vi "SecurityUserInterface.vi"() -> ()   [LabVIEW 2023]
uses:
  Control 2.ctl
  <vilib>/Utility/file.llb/Read Delimited Spreadsheet (string).vi
  <vilib>/Utility/file.llb/Write Delimited Spreadsheet (string).vi
  <vilib>/regexp/Match Regular Expression.xnode
panel:
  in  "LogfileUI":enum32{"Page 1"}(tab)
  out "Table Control":string[][](table)
  in  "LoginMenu":enum32{"Page 1", "Page 2"}(tab)
  in  "OK Button":bool
  in  "Username":string
  in  "Password":string
  out "Current Date & Time":string
  in  "ServerUI":enum32{"Page 2"}(tab)
  in  "Logout":bool
  in  "View Log File":bool
  out "Status1":bool
  out "Status2":bool
  out "Status3":bool
  out "Status4":bool
  out "Status5":bool
  out "Status6":bool
  out "Alarm1":bool
  out "Bypass1":bool
  out "Tamper1":bool
  out "Alarm2":bool
  out "Bypass2":bool
  out "Tamper2":bool
  out "Alarm3":bool
  out "Bypass3":bool
  out "Tamper3":bool
  out "Alarm4":bool
  out "Bypass4":bool
  out "Tamper4":bool
  out "Alarm5":bool
  out "Bypass5":bool
  out "Tamper5":bool
  out "Alarm6":bool
  out "Bypass6":bool
  out "Tamper6":bool
  # "Zone Status Log File"
  # "Login Menu"
  # "Zone Status Indicators Panel"
  # "Green = Normal     Red = Alarm       \nOrange = Tamper   Blue = Bypass"
  # "Zone 1"
  # "Zone 2"
  # "Zone 3"
  # "Zone 4"
  # "Zone 5"
  # "Zone 6"
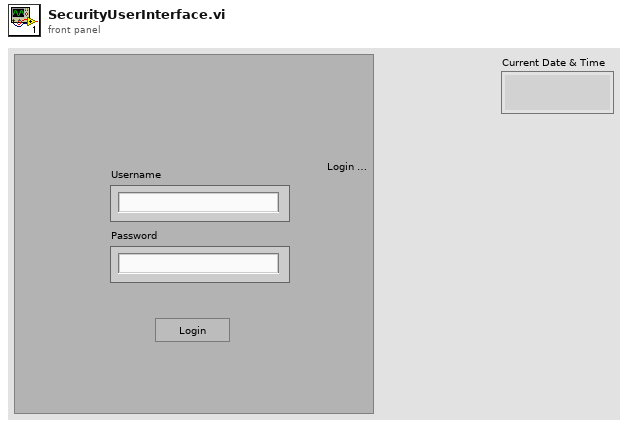
[diagram p1: front panel]
types:
  T1 = typedef "Control 2.ctl" = enum16{"Init", "Wait", "Login", "Logout", "End"}
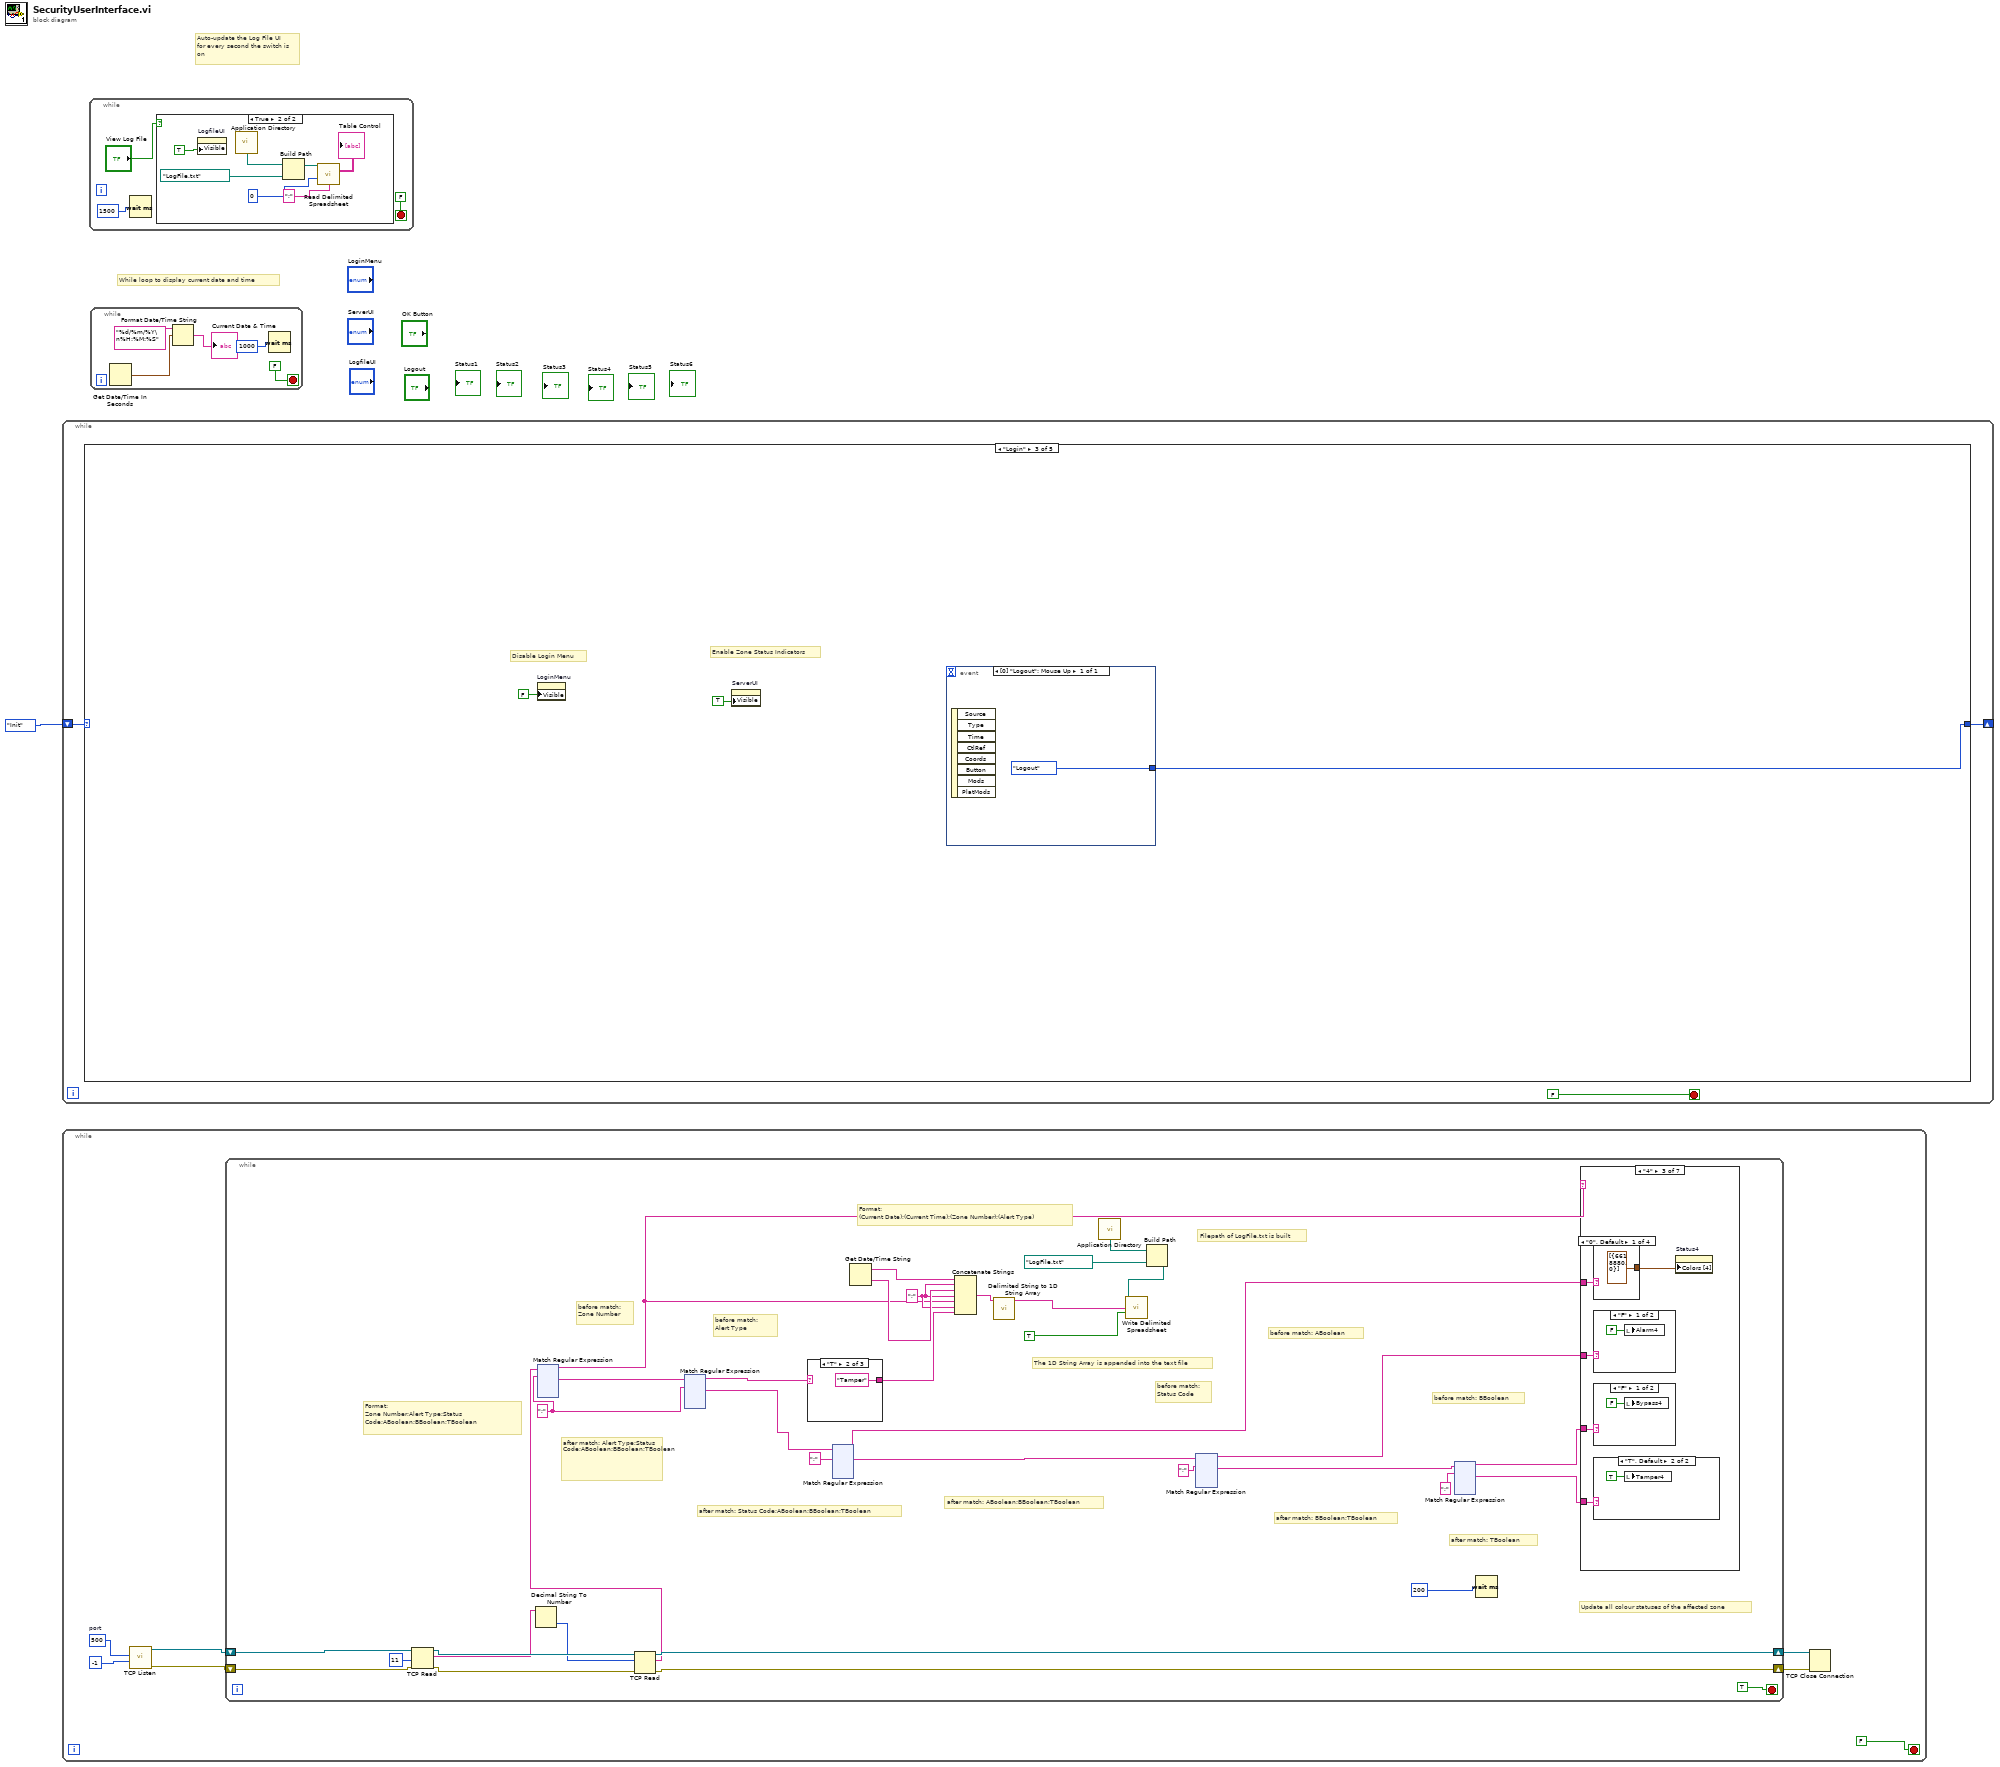
[diagram p0: block diagram]
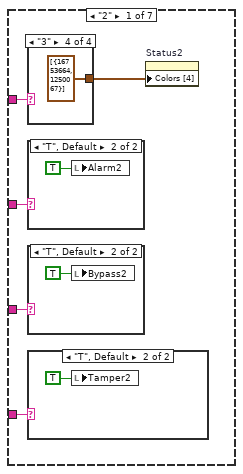
[diagram p2: hidden frame]
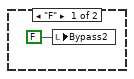
[diagram p3: hidden frame]
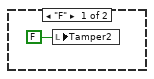
[diagram p4: hidden frame]
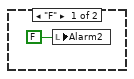
[diagram p5: hidden frame]
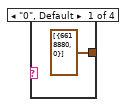
[diagram p6: hidden frame]
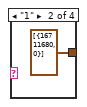
[diagram p7: hidden frame]
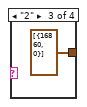
[diagram p8: hidden frame]
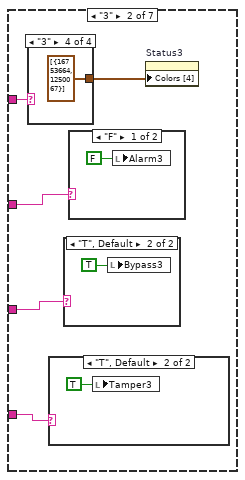
[diagram p9: hidden frame]
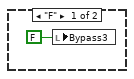
[diagram p10: hidden frame]
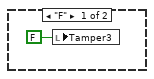
[diagram p11: hidden frame]
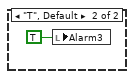
[diagram p12: hidden frame]
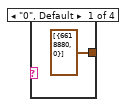
[diagram p13: hidden frame]
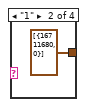
[diagram p14: hidden frame]
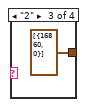
[diagram p15: hidden frame]
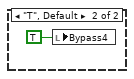
[diagram p16: hidden frame]
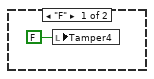
[diagram p17: hidden frame]
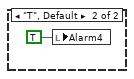
[diagram p18: hidden frame]
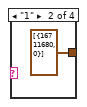
[diagram p19: hidden frame]
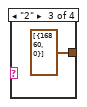
[diagram p20: hidden frame]
diagram:
  # "Auto-update the Log File UI for every second the switch is on"
  # "While loop to display current date and time"
  n1 = while {
    shift-right: [w2] -> _
    shift-left: Control_2."Init" -> [w3]
    stop <- FALSE stop-if-true
    n2 = case shown="\"Login\"" w3 {
      tunnel: [Control_2."Wait" w13 w48 Control_2."Init" Control_2."Init"] -> w2
      frame "Init", Default {
        w8 = cluster{u32, u32}[] [{6618880, 0}] ("Colors [4]")
        w9 = FALSE
        w11 = ""
        # "Enable the Login UI"
        # "Turn off all zone alert LEDs"
        # "Disable Log File Panel"
        # "Initialize all zone statuses to normal state"
        # "Disable Indicator Panel"
        # "Clear Username and Password fields"
        n3 = property on="ServerUI" class="TabCtl (strict)"("Visible"=FALSE) -> ()  [unwired: 2 in, 2 out]
        n4 = property on="LoginMenu" class="TabCtl (strict)"("Visible"=TRUE) -> ()  [unwired: 2 in, 2 out]
        n5 = local write "View Log File"(FALSE ("View Log File")) -> ()
        n6 = local write "Username"(w11) -> ()
        n7 = local write "Password"(w11) -> ()
        n8 = property on="LogfileUI" class="TabCtl (strict)"("Visible"=FALSE) -> ()  [unwired: 2 in, 2 out]
        n9 = property on="Status1" class="Bool (strict)"("Colors [4]"=w8) -> ()  [unwired: 2 in, 2 out]
        n10 = property on="Status2" class="Bool (strict)"("Colors [4]"=w8) -> ()  [unwired: 2 in, 2 out]
        n11 = property on="Status3" class="Bool (strict)"("Colors [4]"=w8) -> ()  [unwired: 2 in, 2 out]
        n12 = property on="Status4" class="Bool (strict)"("Colors [4]"=w8) -> ()  [unwired: 2 in, 2 out]
        n13 = property on="Status5" class="Bool (strict)"("Colors [4]"=w8) -> ()  [unwired: 2 in, 2 out]
        n14 = property on="Status6" class="Bool (strict)"("Colors [4]"=w8) -> ()  [unwired: 2 in, 2 out]
        "Alarm1" <- w9
        "Bypass1" <- w9
        "Tamper1" <- w9
        "Tamper2" <- w9
        "Tamper3" <- w9
        "Tamper4" <- w9
        "Tamper5" <- w9
        "Tamper6" <- w9
        "Alarm4" <- w9
        "Bypass4" <- w9
        "Alarm5" <- w9
        "Bypass5" <- w9
        "Alarm6" <- w9
        "Bypass6" <- w9
        "Alarm3" <- w9
        "Bypass3" <- w9
        "Bypass2" <- w9
        "Alarm2" <- w9
      }
      frame "Wait" {
        n15 = event shown="[0] \"OK Button\": Mouse Up" {
          selector: _ -> [_]
          dyn-events: _ -> [_]
          timeout: _ -> [_]
          tunnel: [w20] -> w13
          event "OK Button": Mouse Up {
            # "Decrement"
            # "Filepath of Users.txt is built"
            # "Array indexing ensures that a username cannot use the password of another user"
            # "Gets an array of usernames"
            # "Gets an array of passwords"
            # "Reads all rows of the Users.txt file into a spreadsheet format with the delimiter ;"
            # "Stops the while loop when it reaches the end of the file, or a matching username has been found"
            n16 = event-data() -> ()  [unwired: 1 in, 8 out]
            n17 = call <vilib>:"Application Directory.vi"() -> ("Application Directory"=w27:path)
            n18 = Build Path(base path=w27, name or relative path="Users.txt") -> (appended path=w26:path)
            n19 = call-poly <vilib>:"Read Delimited Spreadsheet.vi"("file path (dialog if empty)"=w26, "delimiter (\\t)"=";" ("delimiter (\\t)")) -> ("all rows"=w25:string[][])  [unwired: 8 in, 5 out]
            n20 = Index Array "Index Array"(array=w25, index (col)=0) -> (element=w19:string[])  [unwired: 1 in]
            n21 = Array Size(array=w19) -> (size(s)=w18:i32)
            n22 = Index Array "Index Array"(array=w25, index (col)=1) -> (element=w24:string[])  [unwired: 1 in]
            n23 = Decrement(x=w18) -> (x-1=w17:i32)
            n24 = while {
              tunnel: w19 -> [w37] mode=indexing
              tunnel: "Username" -> [w36]
              tunnel: "Password" -> [w35]
              tunnel: w24 -> [w34] mode=indexing
              tunnel: [w33] -> w20
              tunnel: w17 -> [w31]
              i -> [w32]
              stop <- w28 stop-if-true
              n25 = Equal?(x=w36, y=w37) -> (x = y?=w30:bool)
              n26 = Equal?(x=w32, y=w31) -> (x = y?=w29:bool)
              n27 = Or(x=w30, y=w29) -> (x .or. y?=w28:bool)
              n28 = case shown="True" w30 {
                tunnel: w35 -> [_ w42]
                tunnel: w34 -> [_ w43]
                tunnel: [Control_2."Login" w40] -> w33
                frame False {
                  # "When there is no matching username, clear the username field and go back to login"
                  n29 = local write "Username"("") -> ()
                }
                frame True {
                  # "When a matching username is found, check for its corresponding password"
                  n30 = Equal?(x=w42, y=w43) -> (x = y?=w41:bool)
                  n31 = case shown="False" w41 {
                    tunnel: [Control_2."Wait" Control_2."Login"] -> w40
                    frame False {
                      # "When there is no matching password, clear the password field and go back to login"
                      n32 = local write "Password"("") -> ()
                    }
                    frame True {
                      # "Upon entering valid user credentials, a login successful prompt will appear and then redirected to the wait state."
                      n33 = One Button Dialog(message="Login Successful!") -> ()  [unwired: 1 in, 1 out]
                    }
                  }
                }
              }
            }
          }
        }
      }
      frame "Login" {
        # "Disable Login Menu"
        # "Enable Zone Status Indicators"
        n34 = property on="LoginMenu" class="TabCtl (strict)"("Visible"=FALSE) -> ()  [unwired: 2 in, 2 out]
        n35 = property on="ServerUI" class="TabCtl (strict)"("Visible"=TRUE) -> ()  [unwired: 2 in, 2 out]
        n36 = event shown="[0] \"Logout\": Mouse Up" {
          selector: _ -> [_]
          dyn-events: _ -> [_]
          timeout: _ -> [_]
          tunnel: [Control_2."Logout"] -> w48
          event "Logout": Mouse Up {
            n37 = event-data() -> ()  [unwired: 1 in, 8 out]
          }
        }
      }
      frame "Logout" {
      }
      frame "End" {
        # "Ends the program."
        n38 = Stop(stop? (T)=TRUE) -> ()
      }
    }
  }
  n39 = while {
    stop <- FALSE stop-if-true
    w56 = u16 500  # port
    n40 = call <vilib>:"TCP Listen.vi"("timeout ms (wait forever: -1)"=-1, "port"=w56) -> ("error out"=w58:errorcluster, "connection ID"=w59:refnum<k5>)  [unwired: 5 in, 3 out]
    n41 = while {
      shift-right: [w90] -> w61
      shift-left: w59 -> [w88]
      shift-right: [w89] -> w60
      shift-left: w58 -> [w87]
      stop <- TRUE stop-if-true
      w68 = ";"
      w65 = ";" ("regular expression")
      # "before match: ABoolean"
      # "before match: BBoolean"
      # "after match: TBoolean"
      # "after match: BBoolean;TBoolean"
      # "after match: ABoolean;BBoolean;TBoolean"
      # "before match: Status Code"
      # "The 1D String Array is appended into the text file"
      # "Filepath of LogFile.txt is built"
      # "Format:\n(Current Date);(Current Time);(Zone Number);(Alert Type)"
      # "Update all colour statuses of the affected zone"
      # "after match: Status Code;ABoolean;BBoolean;TBoolean"
      # "before match: Alert Type"
      # "after match: Alert Type;Status Code;ABoolean;BBoolean;TBoolean"
      # "before match: Zone Number"
      # "Format:\nZone Number;Alert Type;Status Code;ABoolean;BBoolean;TBoolean"
      n42 = TCP Read(connection ID=w88, bytes to read=11, error in (no error)=w87) -> (connection ID out=w86:refnum<k5>, data out=w85:string, error out=w84:errorcluster)  [unwired: 2 in]
      n43 = Decimal String To Number(string=w85) -> (number=w83:i32)  [unwired: 2 in, 1 out]
      n44 = TCP Read(connection ID=w86, bytes to read=w83, error in (no error)=w84) -> (connection ID out=w90:refnum<k5>, data out=w82:string, error out=w89:errorcluster)  [unwired: 2 in]
      n45 = xnode "Match Regular Expression"("input string"=w82, "regular expression"=w65) -> ("before match"=w63:string, "after match"=w73:string)  [unwired: 4 in, 4 out]
      n46 = xnode "Match Regular Expression"("input string"=w73, "regular expression"=w65) -> ("before match"=w77:string, "after match"=w96:string)  [unwired: 4 in, 4 out]
      n47 = case shown="\"T\"" w77 {
        tunnel: ["Bypass" ("string") "Tamper" ("string") "Alarm" ("string")] -> w81
        frame "B" {
        }
        frame "T" {
        }
        frame "A", Default {
        }
      }
      n48 = xnode "Match Regular Expression"("input string"=w96, "regular expression"=";") -> ("before match"=w91:string, "after match"=w92:string)  [unwired: 4 in, 4 out]
      n49 = Get Date/Time String() -> (date string=w74:string, time string=w80:string)  [unwired: 3 in]
      n50 = Concatenate Strings(w74, w68, w80, w68, w63, w68, w81) -> (w79:string)
      n51 = call <vilib>:"Delimited String to 1D String Array.vi"("delimited string"=w79) -> ("string array"=w78:string[])  [unwired: 10 in]
      n52 = call <vilib>:"Application Directory.vi"() -> ("Application Directory"=w76:path)
      n53 = Build Path(base path=w76, name or relative path=path "LogFile.txt") -> (appended path=w75:path)
      n54 = call-poly <vilib>:"Write Delimited Spreadsheet.vi"("file path (dialog if empty)"=w75, "1D data"=w78, "append to file? (new file:F)"=TRUE) -> ()  [unwired: 11 in, 2 out]
      n55 = xnode "Match Regular Expression"("input string"=w92, "regular expression"=";") -> ("before match"=w94:string, "after match"=w93:string)  [unwired: 4 in, 4 out]
      n56 = xnode "Match Regular Expression"("input string"=w93, "regular expression"=";") -> ("before match"=w95:string, "after match"=w97:string)  [unwired: 4 in, 4 out]
      n57 = Wait (ms)(milliseconds to wait=u32 200) -> ()  [unwired: 1 out]
      n58 = case shown="\"4\"" w63 {
        tunnel: w91 -> [w459 w474 w489 w504 w519 _ w534]
        tunnel: w94 -> [w455 w470 w485 w500 w515 _ w532]
        tunnel: w97 -> [w457 w472 w487 w502 w517 _ w531]
        tunnel: w95 -> [w456 w471 w486 w501 w516 _ w530]
        frame "2" {
          n59 = case shown="\"3\"" w459 {
            tunnel: [cluster{u32, u32}[] [{6618880, 0}] ("Tamper") cluster{u32, u32}[] [{16711680, 0}] ("Tamper") cluster{u32, u32}[] [{16860, 0}] ("Tamper") cluster{u32, u32}[] [{16753664, 1250067}] ("Tamper")] -> w458
            frame "0", Default {
            }
            frame "1" {
            }
            frame "2" {
            }
            frame "3" {
            }
          }
          n60 = case shown="\"T\", Default" w455 {
            frame "F" {
              n61 = local write "Alarm2"(FALSE ("Status1")) -> ()
            }
            frame "T", Default {
              n62 = local write "Alarm2"(TRUE ("Status1")) -> ()
            }
          }
          n63 = case shown="\"T\", Default" w456 {
            frame "F" {
              n64 = local write "Bypass2"(FALSE ("Status1")) -> ()
            }
            frame "T", Default {
              n65 = local write "Bypass2"(TRUE ("Status1")) -> ()
            }
          }
          n66 = case shown="\"T\", Default" w457 {
            frame "F" {
              n67 = local write "Tamper2"(FALSE ("Status1")) -> ()
            }
            frame "T", Default {
              n68 = local write "Tamper2"(TRUE ("Status1")) -> ()
            }
          }
          n69 = property on="Status2" class="Bool (strict)"("Colors [4]"=w458) -> ()  [unwired: 2 in, 2 out]
        }
        frame "3" {
          n70 = case shown="\"3\"" w474 {
            tunnel: [cluster{u32, u32}[] [{6618880, 0}] ("Tamper") cluster{u32, u32}[] [{16711680, 0}] ("Tamper") cluster{u32, u32}[] [{16860, 0}] ("Tamper") cluster{u32, u32}[] [{16753664, 1250067}] ("Tamper")] -> w473
            frame "0", Default {
            }
            frame "1" {
            }
            frame "2" {
            }
            frame "3" {
            }
          }
          n71 = case shown="\"T\", Default" w472 {
            frame "F" {
              n72 = local write "Tamper3"(FALSE ("Status1")) -> ()
            }
            frame "T", Default {
              n73 = local write "Tamper3"(TRUE ("Status1")) -> ()
            }
          }
          n74 = case shown="\"T\", Default" w471 {
            frame "F" {
              n75 = local write "Bypass3"(FALSE ("Status1")) -> ()
            }
            frame "T", Default {
              n76 = local write "Bypass3"(TRUE ("Status1")) -> ()
            }
          }
          n77 = case shown="\"F\"" w470 {
            frame "F" {
              n78 = local write "Alarm3"(FALSE ("Status1")) -> ()
            }
            frame "T", Default {
              n79 = local write "Alarm3"(TRUE ("Status1")) -> ()
            }
          }
          n80 = property on="Status3" class="Bool (strict)"("Colors [4]"=w473) -> ()  [unwired: 2 in, 2 out]
        }
        frame "4" {
          n81 = case shown="\"0\", Default" w489 {
            tunnel: [cluster{u32, u32}[] [{6618880, 0}] ("Tamper") cluster{u32, u32}[] [{16711680, 0}] ("Tamper") cluster{u32, u32}[] [{16860, 0}] ("Tamper") cluster{u32, u32}[] [{16753664, 1250067}] ("Tamper")] -> w488
            frame "0", Default {
            }
            frame "1" {
            }
            frame "2" {
            }
            frame "3" {
            }
          }
          n82 = case shown="\"F\"" w485 {
            frame "F" {
              n83 = local write "Alarm4"(FALSE ("Status1")) -> ()
            }
            frame "T", Default {
              n84 = local write "Alarm4"(TRUE ("Status1")) -> ()
            }
          }
          n85 = case shown="\"F\"" w486 {
            frame "F" {
              n86 = local write "Bypass4"(FALSE ("Status1")) -> ()
            }
            frame "T", Default {
              n87 = local write "Bypass4"(TRUE ("Status1")) -> ()
            }
          }
          n88 = case shown="\"T\", Default" w487 {
            frame "F" {
              n89 = local write "Tamper4"(FALSE ("Status1")) -> ()
            }
            frame "T", Default {
              n90 = local write "Tamper4"(TRUE ("Status1")) -> ()
            }
          }
          n91 = property on="Status4" class="Bool (strict)"("Colors [4]"=w488) -> ()  [unwired: 2 in, 2 out]
        }
        frame "5" {
          n92 = case shown="\"0\", Default" w504 {
            tunnel: [cluster{u32, u32}[] [{6618880, 0}] ("Tamper") cluster{u32, u32}[] [{16711680, 0}] ("Tamper") cluster{u32, u32}[] [{16860, 0}] ("Tamper") cluster{u32, u32}[] [{16753664, 1250067}] ("Tamper")] -> w503
            frame "0", Default {
            }
            frame "1" {
            }
            frame "2" {
            }
            frame "3" {
            }
          }
          n93 = case shown="\"F\"" w500 {
            frame "F" {
              n94 = local write "Alarm5"(FALSE ("Status1")) -> ()
            }
            frame "T", Default {
              n95 = local write "Alarm5"(TRUE ("Status1")) -> ()
            }
          }
          n96 = case shown="\"F\"" w501 {
            frame "F" {
              n97 = local write "Bypass5"(FALSE ("Status1")) -> ()
            }
            frame "T", Default {
              n98 = local write "Bypass5"(TRUE ("Status1")) -> ()
            }
          }
          n99 = case shown="\"F\"" w502 {
            frame "F" {
              n100 = local write "Tamper5"(FALSE ("Status1")) -> ()
            }
            frame "T", Default {
              n101 = local write "Tamper5"(TRUE ("Status1")) -> ()
            }
          }
          n102 = property on="Status5" class="Bool (strict)"("Colors [4]"=w503) -> ()  [unwired: 2 in, 2 out]
        }
        frame "6" {
          n103 = case shown="\"1\"" w519 {
            tunnel: [cluster{u32, u32}[] [{6618880, 0}] ("Tamper") cluster{u32, u32}[] [{16711680, 0}] ("Tamper") cluster{u32, u32}[] [{16860, 0}] ("Tamper") cluster{u32, u32}[] [{16753664, 1250067}] ("Tamper")] -> w518
            frame "0", Default {
            }
            frame "1" {
            }
            frame "2" {
            }
            frame "3" {
            }
          }
          n104 = case shown="\"T\", Default" w515 {
            frame "F" {
              n105 = local write "Alarm6"(FALSE ("Status1")) -> ()
            }
            frame "T", Default {
              n106 = local write "Alarm6"(TRUE ("Status1")) -> ()
            }
          }
          n107 = case shown="\"F\"" w516 {
            frame "F" {
              n108 = local write "Bypass6"(FALSE ("Status1")) -> ()
            }
            frame "T", Default {
              n109 = local write "Bypass6"(TRUE ("Status1")) -> ()
            }
          }
          n110 = case shown="\"F\"" w517 {
            frame "F" {
              n111 = local write "Tamper6"(FALSE ("Status1")) -> ()
            }
            frame "T", Default {
              n112 = local write "Tamper6"(TRUE ("Status1")) -> ()
            }
          }
          n113 = property on="Status6" class="Bool (strict)"("Colors [4]"=w518) -> ()  [unwired: 2 in, 2 out]
        }
        frame "0", Default {
        }
        frame "1" {
          n114 = case shown="\"2\"" w534 {
            tunnel: [cluster{u32, u32}[] [{6618880, 0}] ("Tamper") cluster{u32, u32}[] [{16711680, 0}] ("Tamper") cluster{u32, u32}[] [{16860, 0}] ("Tamper") cluster{u32, u32}[] [{16753664, 1250067}] ("Tamper")] -> w533
            frame "0", Default {
            }
            frame "1" {
            }
            frame "2" {
            }
            frame "3" {
            }
          }
          n115 = case shown="\"T\", Default" w532 {
            frame "F" {
              n116 = local write "Alarm1"(FALSE ("Status1")) -> ()
            }
            frame "T", Default {
              n117 = local write "Alarm1"(TRUE ("Status1")) -> ()
            }
          }
          n118 = case shown="\"T\", Default" w530 {
            frame "F" {
              n119 = local write "Bypass1"(FALSE ("Status1")) -> ()
            }
            frame "T", Default {
              n120 = local write "Bypass1"(TRUE ("Status1")) -> ()
            }
          }
          n121 = case shown="\"F\"" w531 {
            frame "F" {
              n122 = local write "Tamper1"(FALSE ("Status1")) -> ()
            }
            frame "T", Default {
              n123 = local write "Tamper1"(TRUE ("Status1")) -> ()
            }
          }
          n124 = property on="Status1" class="Bool (strict)"("Colors [4]"=w533) -> ()  [unwired: 2 in, 2 out]
        }
      }
    }
    n125 = TCP Close Connection(connection ID=w61, error in (no error)=w60) -> ()  [unwired: 1 in, 2 out]
  }
  n126 = while {
    stop <- FALSE stop-if-true
    n127 = Wait (ms)(milliseconds to wait=u32 1500) -> ()  [unwired: 1 out]
    n128 = case shown="True" "View Log File" {
      frame False {
        n129 = property on="LogfileUI" class="TabCtl (strict)"("Visible"=FALSE) -> ()  [unwired: 2 in, 2 out]
      }
      frame True {
        n130 = property on="LogfileUI" class="TabCtl (strict)"("Visible"=TRUE) -> ()  [unwired: 2 in, 2 out]
        n131 = call <vilib>:"Application Directory.vi"() -> ("Application Directory"=w795:path)
        n132 = Build Path(base path=w795, name or relative path=path "LogFile.txt") -> (appended path=w793:path)
        n133 = call-poly <vilib>:"Read Delimited Spreadsheet.vi"("file path (dialog if empty)"=w793, "max characters/row  (no limit:0)"=0, "delimiter (\\t)"=";" ("delimiter (\\t)")) -> ("all rows"=→"Table Control":string[][])  [unwired: 7 in, 5 out]
      }
    }
  }
  n134 = while {
    stop <- FALSE stop-if-true
    n135 = Get Date/Time In Seconds() -> (seconds since 1Jan1904=w800:timestamp)
    n136 = Format Date/Time String(time format string (%c)="%d/%m/%Y\n%H:%M:%S", seconds (now)=w800) -> (date/time string=→"Current Date & Time":string)  [unwired: 1 in]
    n137 = Wait (ms)(milliseconds to wait=u32 1000) -> ()  [unwired: 1 out]
  }
